vi "Finalize Spawn.vi"(8 "Error in":errorcluster, 10 "Attributes":refnum<data-value>, 11 "Actor in":refnum<class "Actor.lvclass">) -> (0 "Error out":errorcluster, 3 "Actor out":refnum<class "Actor.lvclass">)   [LabVIEW 2020, in "jettl.lvlib" / "Actor.lvclass"]
uses:
  Actor.lvclass
  Msg/Msg.lvclass
  Transport/Transport.lvclass
  Actor Attributes.ctl
  jettl.lvlib
  Msgs.ctl
  Unified Layer.ctl
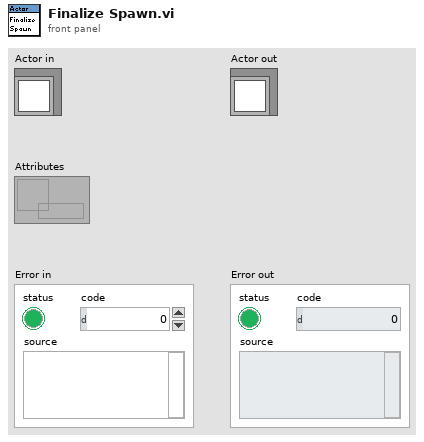
[diagram p1: front panel]
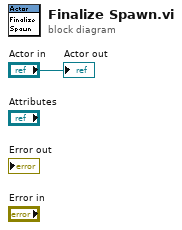
[diagram p0: block diagram]
diagram:
  "Actor out" <- "Actor in"
